vi "Update Tracking Table.vi"(0 "Tracking In":string[][](array[string]), 5 "TrackingRowsSel":i32[](array[numeric]), 7 "CalChannelsArray":string[][](array[string]), 9 "Tolerancing Bundle":T1(array[cluster]), 11 "CalState":i32, 13 "TrackingTableColors In":i32[][](array[numeric])) -> (4 "Tracking Out":string[][](array[string]), 15 "TrackingTableColors Out":i32[][](array[numeric]))   [LabVIEW 2019]
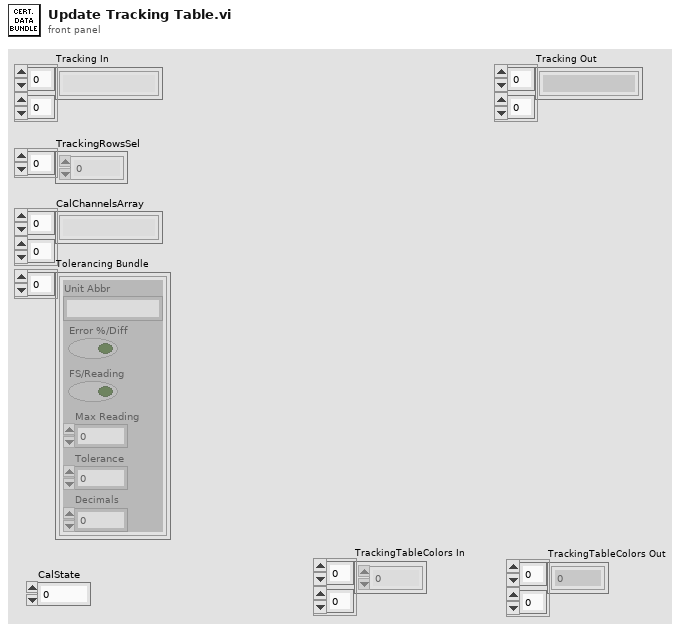
[diagram p1: front panel]
types:
  T1 = cluster{"Unit Abbr":string, "Error %/Diff":bool, "FS/Reading":bool, "Max Reading":dbl, "Tolerance":dbl, "Decimals":i16}[]
  T2 = cluster{"Unit Abbr":string, "Error %/Diff":bool, "FS/Reading":bool, "Max Reading":dbl, "Tolerance":dbl, "Decimals":i16}
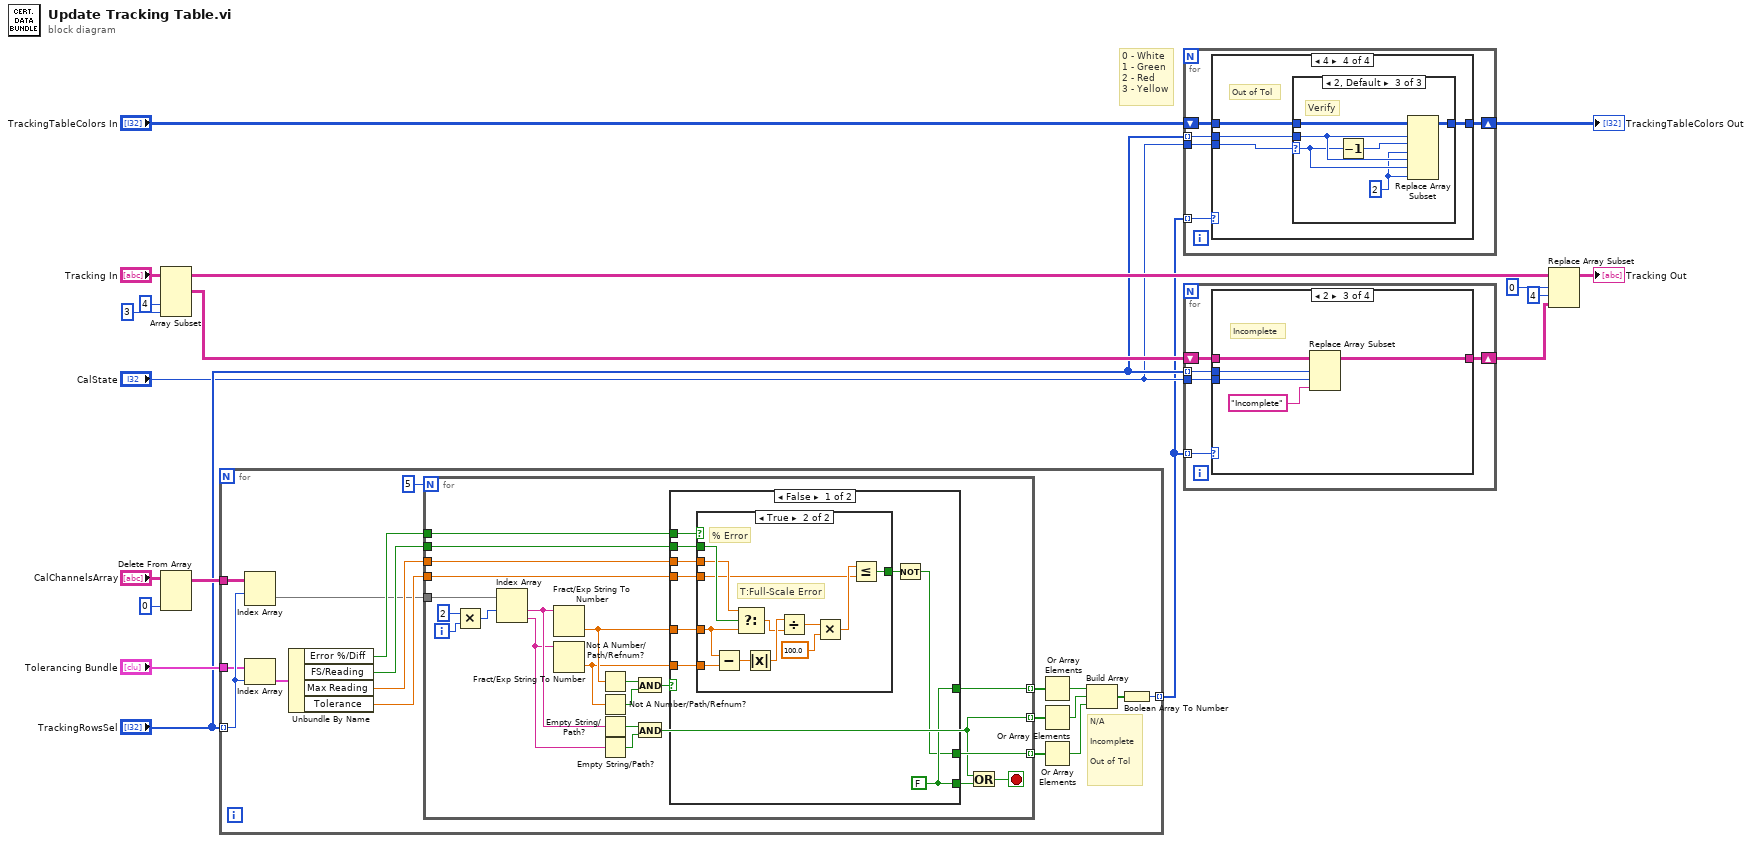
[diagram p0: block diagram]
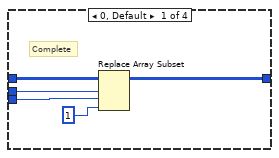
[diagram p2: hidden frame]
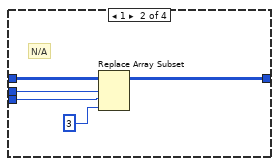
[diagram p3: hidden frame]
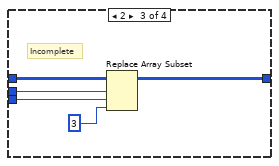
[diagram p4: hidden frame]
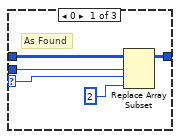
[diagram p5: hidden frame]
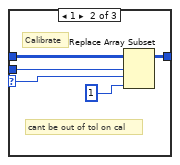
[diagram p6: hidden frame]
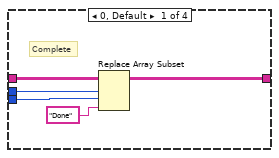
[diagram p7: hidden frame]
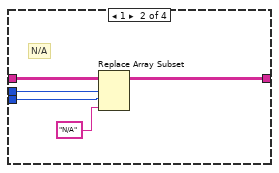
[diagram p8: hidden frame]
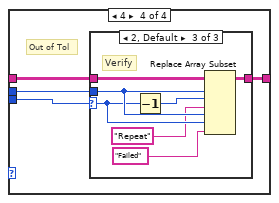
[diagram p9: hidden frame]
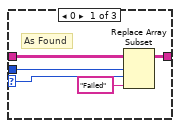
[diagram p10: hidden frame]
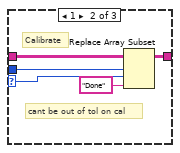
[diagram p11: hidden frame]
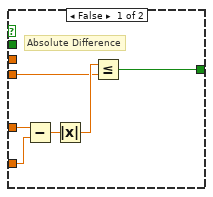
[diagram p12: hidden frame]
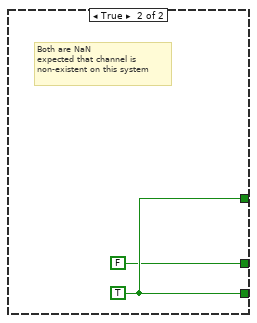
[diagram p13: hidden frame]
diagram:
  # "0 - White\n1 - Green\n2 - Red\n3 - Yellow"
  n1 = Array Subset(array="Tracking In", index (col)=4 ("index"), length (col)=3 ("length")) -> (w7:string[][])  [unwired: 2 in]
  n2 = Delete From Array(array="CalChannelsArray", index (col)=0 ("disabled index (col)")) -> (array with subset deleted=w15:string[][])  [unwired: 2 in, 1 out]
  n3 = for {
    tunnel: w15 -> [w28]
    tunnel: "Tolerancing Bundle" -> [w29]
    tunnel: "TrackingRowsSel" -> [w30] mode=indexing
    tunnel: [w18] -> w2 mode=indexing
    # "N/A\n\nIncomplete\n\nOut of Tol"
    n4 = Index Array(array=w28, index (row)=w30) -> (element=w27:string[])  [unwired: 1 in]
    n5 = Index Array(array=w29, index=w30) -> (element=w26:T2)
    n6 = Unbundle By Name(w26) -> ("Error %/Diff"=w34:bool, "FS/Reading"=w33:bool, "Max Reading"=w32:dbl, "Tolerance"=w31:dbl)
    n7 = for {
      N: 5 -> [_]
      tunnel: w27 -> [w56]
      tunnel: w34 -> [w49]
      tunnel: w33 -> [w48]
      tunnel: w32 -> [w47]
      tunnel: w31 -> [w46]
      tunnel: [w44] -> w25 mode=indexing
      tunnel: [w36] -> w24 mode=indexing
      tunnel: [w43] -> w23 mode=indexing
      i -> [w45]
      stop <- w37 stop-if-true
      n8 = Multiply(x=2, y=w45) -> (x*y=w55:i32)
      n9 = Index Array(array=w56, index #1=w55) -> (element #1=w42:string, element #2=w41:string)  [unwired: 1 in]
      n10 = Fract/Exp String To Number(string=w42) -> (number=w51:dbl)  [unwired: 3 in, 1 out]
      n11 = Fract/Exp String To Number(string=w41) -> (number=w50:dbl)  [unwired: 3 in, 1 out]
      n12 = Not A Number/Path/Refnum?(number/path/refnum=w51) -> (NaN/Path/Refnum?=w54:bool)
      n13 = Not A Number/Path/Refnum?(number/path/refnum=w50) -> (NaN/Path/Refnum?=w53:bool)
      n14 = Empty String/Path?(string/path=w42) -> (empty?=w40:bool)
      n15 = Empty String/Path?(string/path=w41) -> (empty?=w39:bool)
      n16 = And(x=w54, y=w53) -> (x .and. y?=w52:bool)
      n17 = And(x=w40, y=w39) -> (x .and. y?=w36:bool)
      n18 = case shown="False" w52 {
        tunnel: w51 -> [w64 _]
        tunnel: w50 -> [w63 _]
        tunnel: w49 -> [w65 _]
        tunnel: w48 -> [w66 _]
        tunnel: w47 -> [w61 _]
        tunnel: w46 -> [w62 _]
        tunnel: [w60 w86] -> w38
        tunnel: [w60 w86] -> w44
        tunnel: [w58 FALSE] -> w43
        frame False {
          w60 = FALSE
          n19 = case shown="True" w65 {
            tunnel: w66 -> [_ w79]
            tunnel: w64 -> [w72 w77]
            tunnel: w63 -> [w71 w84]
            tunnel: w62 -> [w68 w74]
            tunnel: w61 -> [_ w78]
            tunnel: [w67 w73] -> w59
            frame False {
              # "Absolute Difference"
              n20 = Subtract(x=w72, y=w71) -> (x-y=w70:dbl)
              n21 = Absolute Value(x=w70) -> (abs(x)=w69:dbl)
              n22 = Less Or Equal?(x=w69, y=w68) -> (x <= y?=w67:bool)
            }
            frame True {
              # "T:Full-Scale Error"
              # "% Error"
              n23 = Subtract(x=w77, y=w84) -> (x-y=w83:dbl)
              n24 = Select(t=w78, s=w79, f=w77) -> (s? t:f=w76:dbl)
              n25 = Absolute Value(x=w83) -> (abs(x)=w82:dbl)
              n26 = Divide(x=w82, y=w76) -> (x/y=w81:dbl)
              n27 = Multiply(x=w81, y=100.0) -> (x*y=w75:dbl)
              n28 = Less Or Equal?(x=w75, y=w74) -> (x <= y?=w73:bool)
            }
          }
          n29 = Not(x=w59) -> (.not. x?=w58:bool)
        }
        frame True {
          w86 = TRUE
          # "Both are NaN\nexpected that channel is\nnon-existent on this system"
        }
      }
      n30 = Or(x=w36, y=w38) -> (x .or. y?=w37:bool)
    }
    n31 = Or Array Elements(Boolean array=w25) -> (logical OR=w22:bool)
    n32 = Or Array Elements(Boolean array=w24) -> (logical OR=w21:bool)
    n33 = Or Array Elements(Boolean array=w23) -> (logical OR=w20:bool)
    n34 = Build Array(w22, w21, w20) -> (w19:bool[])
    n35 = Boolean Array To Number(Boolean array=w19) -> (number=w18:u32)
  }
  n36 = for {
    tunnel: "TrackingRowsSel" -> [w89] mode=indexing
    shift-right: [w90] -> w1
    shift-left: "TrackingTableColors In" -> [w91]
    tunnel: w2 -> [w87] mode=indexing
    tunnel: "CalState" -> [w88]
    n37 = case shown="4" w87 {
      tunnel: w91 -> [w96 w101 w106 w110]
      tunnel: [w95 w100 w105 w109] -> w90
      tunnel: w89 -> [w94 w99 w104 w108]
      tunnel: w88 -> [w93 w98 w103 w107]
      frame 0, Default {
        # "Complete"
        n38 = Replace Array Subset(array=w96, new element=1, index (row)=w94, index (col)=w93) -> (w95:i32[][])
      }
      frame 1 {
        # "N/A"
        n39 = Replace Array Subset(array=w101, new element=3 ("new element/subarray"), index (row)=w99, index (col)=w98) -> (w100:i32[][])
      }
      frame 2 {
        # "Incomplete"
        n40 = Replace Array Subset(array=w106, new element=3, index (row)=w104, index (col)=w103) -> (w105:i32[][])
      }
      frame 4 {
        # "Out of Tol"
        n41 = case shown="2, Default" w107 {
          selector: w107 -> [w112 w117 w123]
          tunnel: w110 -> [w115 w120 w126]
          tunnel: [w114 w119 w125] -> w109
          tunnel: w108 -> [w113 w118 w124]
          frame 0 {
            # "As Found"
            n42 = Replace Array Subset(array=w115, new element=2, index (row)=w113, index (col)=w112) -> (w114:i32[][])
          }
          frame 1 {
            # "cant be out of tol on cal"
            # "Calibrate"
            n43 = Replace Array Subset(array=w120, new element=1 ("new element/subarray"), index (row)=w118, index (col)=w117) -> (w119:i32[][])
          }
          frame 2, Default {
            w121 = 2
            # "Verify"
            n44 = Decrement(x=w123) -> (x-1=w122:i32)
            n45 = Replace Array Subset(array=w126, new element #1=w121, index (row) #1=w124, index (col) #1=w122, new element #2=w121, index (row) #2=w124, index (col) #2=w123) -> (w125:i32[][])
          }
        }
      }
    }
  }
  "TrackingTableColors Out" <- w1
  n46 = for {
    tunnel: "TrackingRowsSel" -> [w129] mode=indexing
    shift-right: [w130] -> w8
    shift-left: w7 -> [w131]
    tunnel: w2 -> [w127] mode=indexing
    tunnel: "CalState" -> [w128]
    n47 = case shown="2" w127 {
      tunnel: w131 -> [w136 w141 w146 w150]
      tunnel: [w135 w140 w145 w149] -> w130
      tunnel: w129 -> [w134 w139 w144 w148]
      tunnel: w128 -> [w133 w137 w143 w147]
      frame 0, Default {
        # "Complete"
        n48 = Replace Array Subset(array=w136, new element="Done" ("new element/subarray"), index (row)=w134, index (col)=w133) -> (w135:string[][])
      }
      frame 1 {
        # "N/A"
        n49 = Replace Array Subset(array=w141, new element="N/A", index (row)=w139, index (col)=w137) -> (w140:string[][])
      }
      frame 2 {
        # "Incomplete"
        n50 = Replace Array Subset(array=w146, new element="Incomplete" ("new element/subarray"), index (row)=w144, index (col)=w143) -> (w145:string[][])
      }
      frame 4 {
        # "Out of Tol"
        n51 = case shown="2, Default" w147 {
          selector: w147 -> [w151 w157 w164]
          tunnel: w150 -> [w155 w160 w167]
          tunnel: [w154 w159 w166] -> w149
          tunnel: w148 -> [w153 w158 w165]
          frame 0 {
            # "As Found"
            n52 = Replace Array Subset(array=w155, new element="Failed" ("new element/subarray"), index (row)=w153, index (col)=w151) -> (w154:string[][])
          }
          frame 1 {
            # "cant be out of tol on cal"
            # "Calibrate"
            n53 = Replace Array Subset(array=w160, new element="Done" ("new element/subarray"), index (row)=w158, index (col)=w157) -> (w159:string[][])
          }
          frame 2, Default {
            # "Verify"
            n54 = Decrement(x=w164) -> (x-1=w163:i32)
            n55 = Replace Array Subset(array=w167, new element #1="Repeat", index (row) #1=w165, index (col) #1=w163, new element #2="Failed", index (row) #2=w165, index (col) #2=w164) -> (w166:string[][])
          }
        }
      }
    }
  }
  n56 = Replace Array Subset(array="Tracking In", new element=w8, index (row)=0 ("disabled index (row)"), index (col)=4 ("disabled index (col)")) -> (→"Tracking Out":string[][])
